vi "PH_Cont-601k_PSU.evt Call Set Voltage.vi"(0 "i ref in":refnum<vi>, 1 "Instance name":string="N/A", 4 "Voltage to set [V]":u16, 5 "error in":errorcluster, 6 "Limits [V]":cluster{"Lower":dbl, "Upper":dbl}) -> (14 "i ref out":refnum<vi>, 19 "error out":errorcluster)   [LabVIEW 2014, in "PH_Cont-601k_PSU.lvlib"]
doc: "This VI calls an event by a simple call."
uses:
  PH_Cont-601k_PSU.lvlib
  CSCore/CSSystem/CoreLib/CoreLib.short 2 byte array.vi
  CSCore/BaseProcess/BaseProcess.lvlib
  CSCore/CSSystem/CoreLib/CoreLib.lvlib
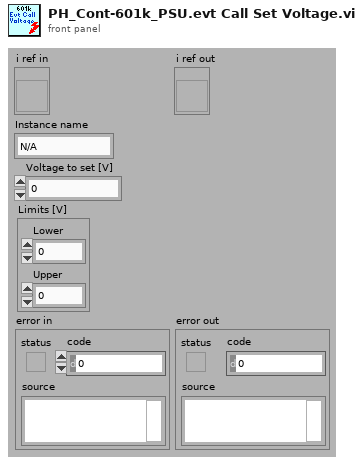
[diagram p1: front panel]
types:
  T1 = typedef "CoreDefs.rawDataType.ctl" = i8[]
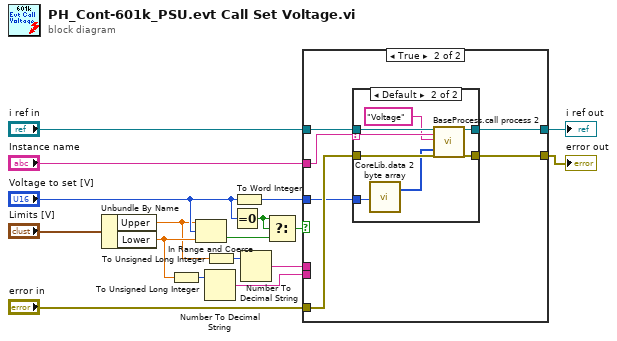
[diagram p0: block diagram]
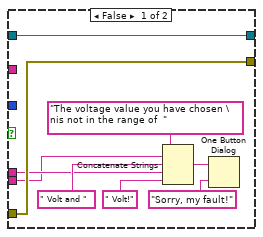
[diagram p2: hidden frame]
diagram:
  n1 = Unbundle By Name("Limits [V]") -> ("Upper"=w1:dbl, "Lower"=w6:dbl)
  n2 = To Unsigned Long Integer(number=w6) -> (unsigned 32bit integer=w3:u32)
  n3 = In Range and Coerce(upper limit=w1, x="Voltage to set [V]", lower limit=w6) -> (In Range?=w10:bool)  [unwired: 1 out]
  n4 = Number To Decimal String(number=w3) -> (decimal integer string=w5:string)  [unwired: 1 in]
  n5 = To Unsigned Long Integer(number=w1) -> (unsigned 32bit integer=w2:u32)
  n6 = Equal To 0?(x="Voltage to set [V]") -> (x = 0?=w11:bool)
  n7 = To Word Integer(number="Voltage to set [V]") -> (16bit integer=w4:i16)
  n8 = Number To Decimal String(number=w2) -> (decimal integer string=w7:string)  [unwired: 1 in]
  n9 = Select(t=w11, s=w11, f=w10) -> (s? t:f=w9:bool)
  n10 = case shown="True" w9 {
    tunnel: [w25 w29] -> w17
    tunnel: "Instance name" -> [_ w32]
    tunnel: "error in" -> [w25 w30]
    tunnel: [w26 w28] -> w14
    tunnel: "i ref in" -> [w26 w31]
    tunnel: w4 -> [_ w27]
    tunnel: w7 -> [w19 _]
    tunnel: w5 -> [w18 _]
    frame False {
      n11 = Concatenate Strings("The voltage value you have chosen \nis not in the range of  ", w18, " Volt and ", w19, " Volt!") -> (w24:string)
      n12 = One Button Dialog(message=w24, button name ("OK")="Sorry, my fault!") -> ()  [unwired: 1 out]
    }
    frame True {
      n13 = case shown="Default" w32 {
        selector: w32 -> [_ w38]
        tunnel: [w33 w42] -> w29
        tunnel: w30 -> [w33 w41]
        tunnel: [w34 w40] -> w28
        tunnel: w31 -> [w34 w39]
        tunnel: w27 -> [_ w35]
        frame "", "N/A" {
        }
        frame Default {
          n14 = call-poly "CoreLib.data 2 byte array.vi"("i16"=w35) -> ("byteArray out"=w36:T1)  [unwired: 18 in]
          n15 = call "BaseProcess.call process 2.vi"("i ref in"=w39, "Object"=w38, "Selector"="Voltage", "Data"=w36, "error in (no error)"=w41) -> ("i ref out"=w40:refnum<vi>, "error out"=w42:errorcluster)  [unwired: 13 in]
        }
      }
    }
  }
  "error out" <- w17
  "i ref out" <- w14
